vi "Coral Configuration.vi"() -> (2 "Algae Config":T2={"Setpoint Configs"=[{"Position Setpoint"=0.0, "Algae State"=enum."Idle", "Power Output"=0.0}, {"Position Setpoint"=5.0, "Algae State"=enum."Intake/Outtake", "Power Output"=-0.5}, {"Position Setpoint"=2.0, "Algae State"=enum."Intake/Outtake", "Power Output"=0.3}, {"Position Setpoint"=2.0, "Algae State"=enum."Stow", "Power Output"=-0.9}]}, 3 "Coral Config":T4={"Setpoint Configs"=[{"Scoring Setpoint"=enum."Trough", "Position Setpoint"=-9.0, "Trapezoid"=[-0.0, -40.0, -80.0, -120.0, -160.0, -200.0, -240.0, -280.0, -320.0, -360.0, -400.0, -440.0, -480.0, -520.0, -560.0, -600.0, -640.0, -680.0, -720.0, -760.0, -800.0, -840.0, -880.0, -920.0, -960.0, -1000.0, -960.0, -919.9999999999999, -879.9999999999999, -840.0000000000001, -800.0, -760.0, -720.0, -680.0, -639.9999999999999, -600.0000000000001, -560.0, -520.0, -480.0, -440.0, -399.9999999999999, -360.0000000000001, -320.0000000000001, -280.0, -240.0, -200.0, -159.9999999999999, -120.00000000000011, -80.00000000000011, -40.0, 0.0], "Score Power"=0.3}, {"Scoring Setpoint"=enum."L2", "Position Setpoint"=-9.7, "Trapezoid"=[], "Score Power"=0.5}, {"Scoring Setpoint"=enum."L3", "Position Setpoint"=-19.5, "Trapezoid"=[], "Score Power"=0.5}, {"Scoring Setpoint"=enum."L4", "Position Setpoint"=-34.9, "Trapezoid"=[], "Score Power"=0.9}, {"Scoring Setpoint"=enum."Default", "Position Setpoint"=0.0, "Trapezoid"=[], "Score Power"=0.0}]})   [LabVIEW 2023]
uses:
  Scoring Levels.ctl
  Algae Setpoint.ctl
panel:
  in  "Algae Intake Value":T2={"Setpoint Configs"=[{"Position Setpoint"=0.0, "Algae State"=enum."Idle", "Power Output"=0.0}, {"Position Setpoint"=5.0, "Algae State"=enum."Intake/Outtake", "Power Output"=-0.5}, {"Position Setpoint"=2.0, "Algae State"=enum."Intake/Outtake", "Power Output"=0.3}, {"Position Setpoint"=2.0, "Algae State"=enum."Stow", "Power Output"=-0.9}]}
  in  "Coral Config L3 Default":T4={"Setpoint Configs"=[{"Scoring Setpoint"=enum."Trough", "Position Setpoint"=-2.3, "Trapezoid"=[0.0, 80.0, 160.0, 240.0, 320.0, 400.0, 480.0, 560.0, 640.0, 720.0, 800.0, 880.0, 960.0, 960.0, 879.9999999999999, 800.0, 720.0, 639.9999999999999, 560.0, 480.0, 399.9999999999999, 320.0000000000001, 240.0, 159.9999999999999, 80.00000000000011, 0.0], "Score Power"=0.3}, {"Scoring Setpoint"=enum."L2", "Position Setpoint"=-3.5, "Trapezoid"=[0.0, 80.0, 160.0, 240.0, 320.0, 400.0, 480.0, 560.0, 640.0, 720.0, 800.0, 720.0000238418579, 640.0000238418579, 560.0000238418579, 480.0000238418578, 400.00002384185797, 320.0000238418579, 240.0000238418578, 160.0000238418579, 80.00002384185791, 0.0], "Score Power"=0.3}, {"Scoring Setpoint"=enum."L3", "Position Setpoint"=-7.0, "Trapezoid"=[], "Score Power"=0.2}, {"Scoring Setpoint"=enum."L4", "Position Setpoint"=-12.15, "Trapezoid"=[-0.0, -80.0, -160.0, -240.0, -320.0, -400.0, -480.0, -560.0, -640.0, -720.0, -800.0, -880.0, -960.0, -1040.0, -1120.0, -1200.0, -1280.0, -1247.6810359954834, -1167.6810359954834, -1087.6810359954834, -1007.6810359954833, -927.6810359954834, -847.6810359954834, -767.6810359954833, -687.6810359954835, -607.6810359954834, -527.6810359954833, -447.6810359954833, -367.68103599548317, -287.6810359954835, -207.6810359954834, -127.6810359954834, -47.6810359954834, 0.0], "Score Power"=0.9}]}
  in  "Ground Intake Coral":T2={"Setpoint Configs"=[{"Position Setpoint"=0.0, "Algae State"=enum."Idle", "Power Output"=0.0}, {"Position Setpoint"=8.5, "Algae State"=enum."Intake/Outtake", "Power Output"=-0.6}, {"Position Setpoint"=3.0, "Algae State"=enum."Intake/Outtake", "Power Output"=0.6}, {"Position Setpoint"=0.5, "Algae State"=enum."Stow", "Power Output"=-0.6}]}
  in  "Coral Config Trusted Values":T4={"Setpoint Configs"=[{"Scoring Setpoint"=enum."Trough", "Position Setpoint"=-9.0, "Trapezoid"=[-0.0, -40.0, -80.0, -120.0, -160.0, -200.0, -240.0, -280.0, -320.0, -360.0, -400.0, -440.0, -480.0, -520.0, -560.0, -600.0, -640.0, -680.0, -720.0, -760.0, -800.0, -840.0, -880.0, -920.0, -960.0, -1000.0, -960.0, -919.9999999999999, -879.9999999999999, -840.0000000000001, -800.0, -760.0, -720.0, -680.0, -639.9999999999999, -600.0000000000001, -560.0, -520.0, -480.0, -440.0, -399.9999999999999, -360.0000000000001, -320.0000000000001, -280.0, -240.0, -200.0, -159.9999999999999, -120.00000000000011, -80.00000000000011, -40.0, 0.0], "Score Power"=0.3}, {"Scoring Setpoint"=enum."L2", "Position Setpoint"=-9.7, "Trapezoid"=[], "Score Power"=0.5}, {"Scoring Setpoint"=enum."L3", "Position Setpoint"=-19.5, "Trapezoid"=[], "Score Power"=0.5}, {"Scoring Setpoint"=enum."L4", "Position Setpoint"=-34.9, "Trapezoid"=[], "Score Power"=0.9}, {"Scoring Setpoint"=enum."Default", "Position Setpoint"=0.0, "Trapezoid"=[], "Score Power"=0.0}]}
  # "L2:  -250 or -100 test\nL3: -450\nL4:-755"
  # "old values"
  # "-2.6"
  # "sp: 0.5"
  # "-4"
  # "sp: 0.5"
  # "-7.7"
  # "-600?"
  # "sp: 0.9"
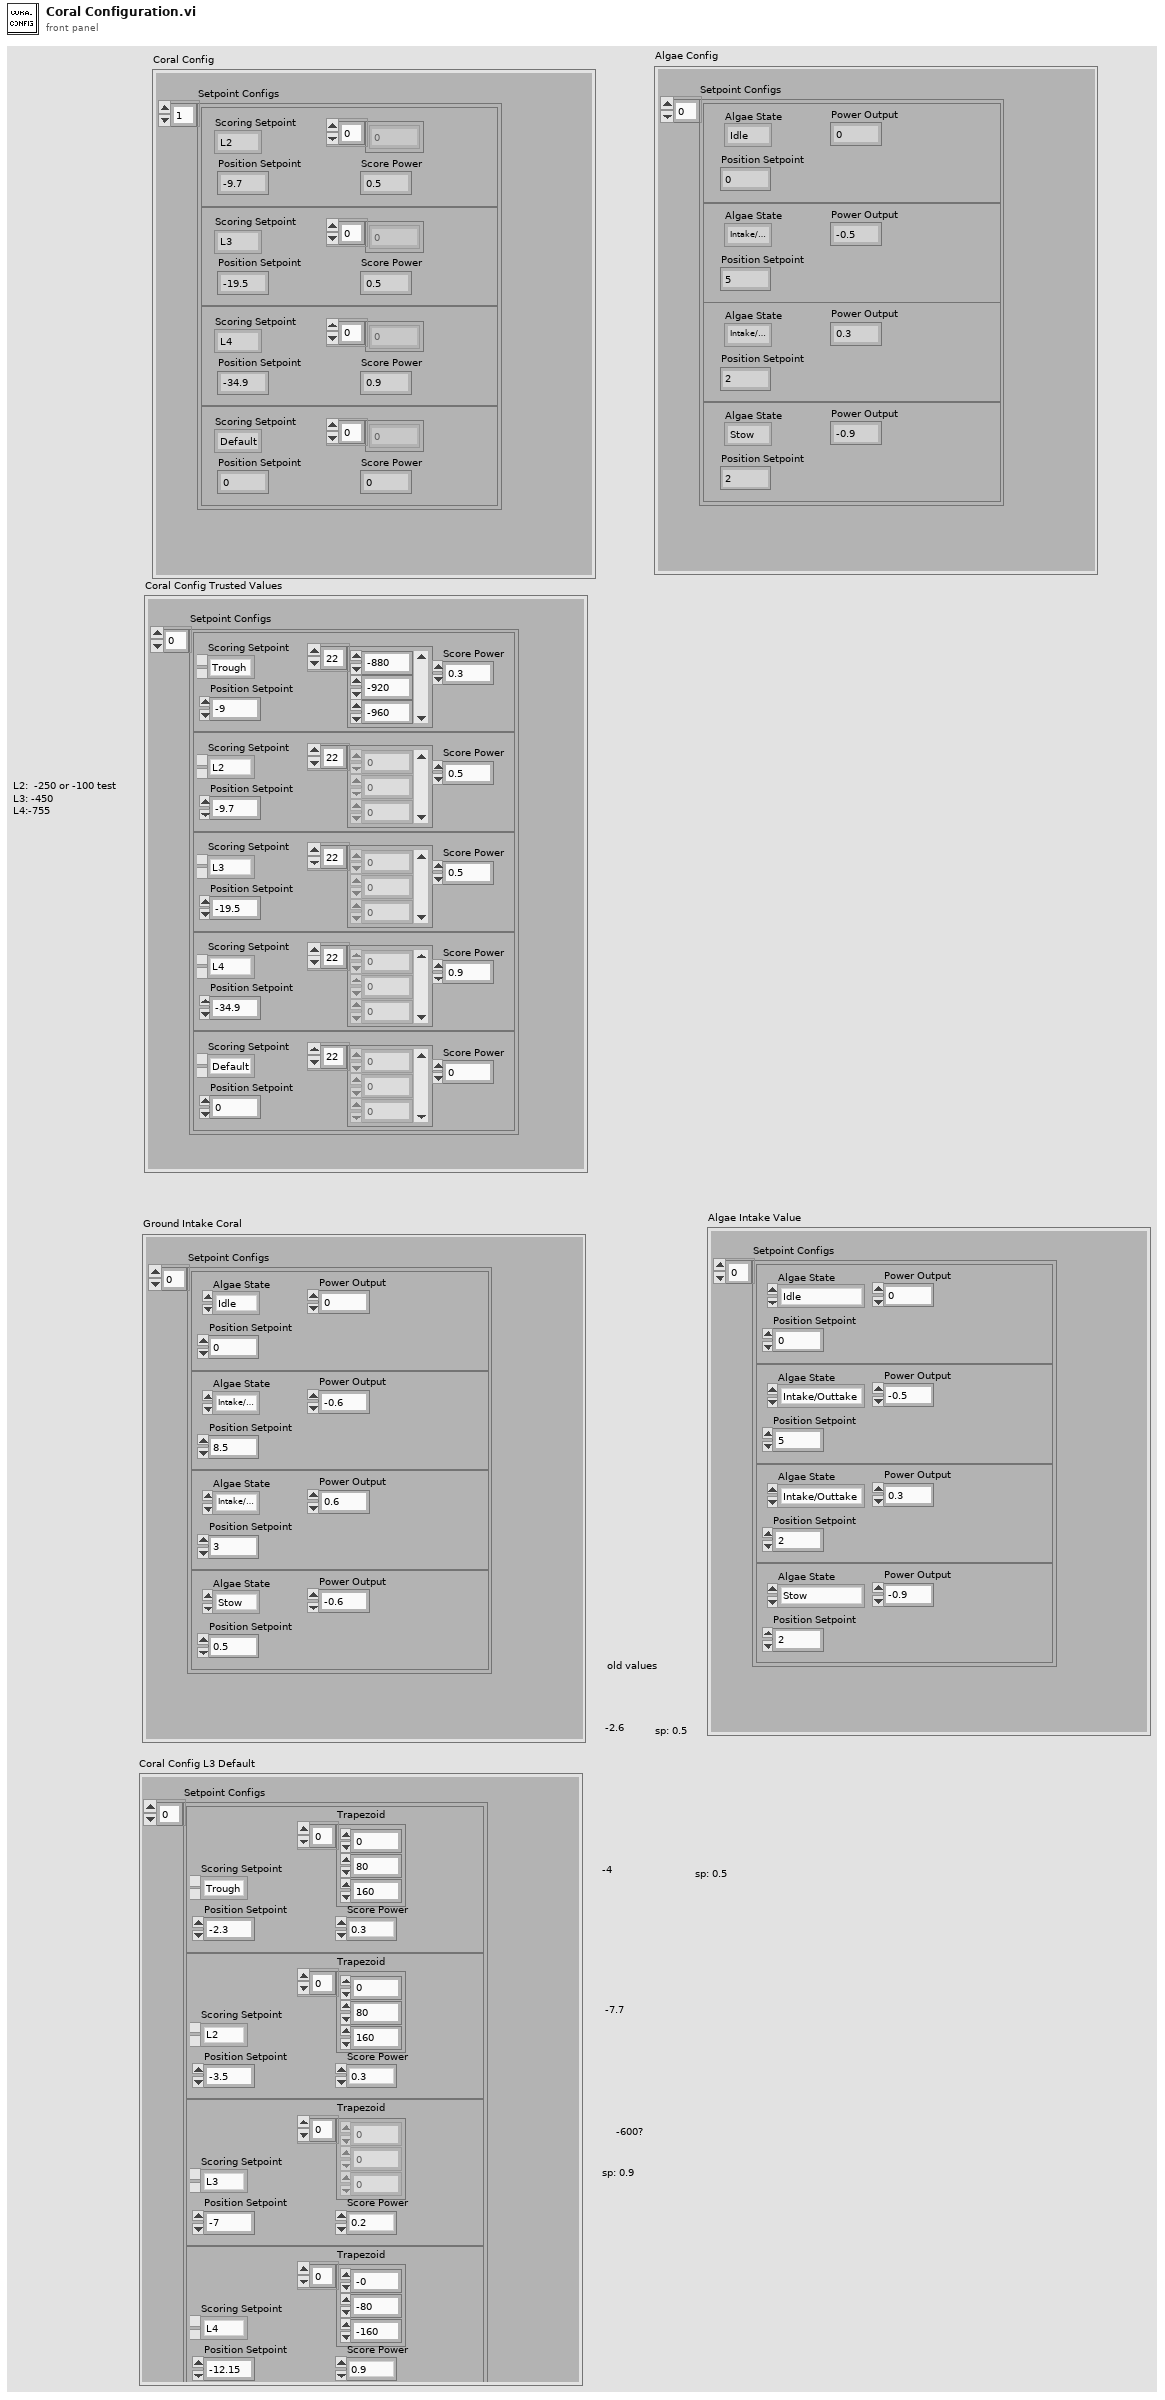
[diagram p1: front panel]
types:
  T1 = typedef "Algae Setpoint.ctl" = enum16{"Idle", "Stow", "Intake/Outtake"}
  T2 = cluster{"Setpoint Configs":cluster{"Position Setpoint":dbl, "Algae State":T1, "Power Output":dbl}[]}
  T3 = typedef "Scoring Levels.ctl" = enum16{"Trough", "L2", "L3", "L4", "Default"}
  T4 = cluster{"Setpoint Configs":cluster{"Scoring Setpoint":T3, "Position Setpoint":dbl, "Trapezoid":dbl[], "Score Power":dbl}[]}
  T5 = cluster{"Setpoint Configs":cluster{"Scoring Setpoint":T3, "Position Setpoint":dbl, "Trapezoid":dbl[]}[]}
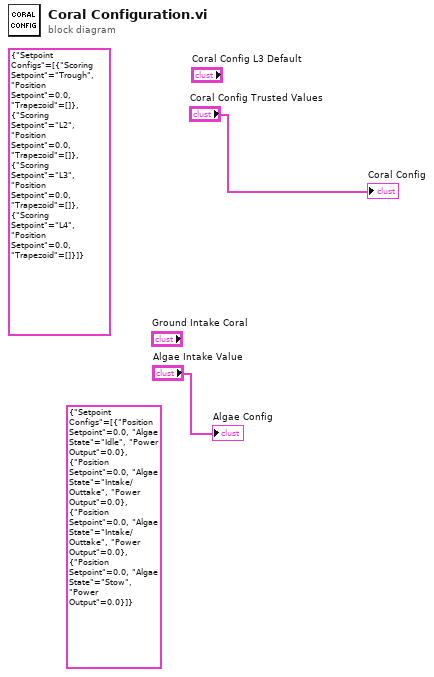
[diagram p0: block diagram]
diagram:
  (unwired) T2 {"Setpoint Configs"=[{"Position Setpoint"=0.0, "Algae State"=enum."Idle", "Power Output"=0.0}, {"Position Setpoint"=0.0, "Algae State"=enum."Intake/Outtake", "Power Output"=0.0}, {"Position Setpoint"=0.0, "Algae State"=enum."Intake/Outtake", "Power Output"=0.0}, {"Position Setpoint"=0.0, "Algae State"=enum."Stow", "Power Output"=0.0}]} ("Algae Config")
  (unwired) T5 {"Setpoint Configs"=[{"Scoring Setpoint"=enum."Trough", "Position Setpoint"=0.0, "Trapezoid"=[]}, {"Scoring Setpoint"=enum."L2", "Position Setpoint"=0.0, "Trapezoid"=[]}, {"Scoring Setpoint"=enum."L3", "Position Setpoint"=0.0, "Trapezoid"=[]}, {"Scoring Setpoint"=enum."L4", "Position Setpoint"=0.0, "Trapezoid"=[]}]} ("Coral Config")
  "Coral Config" <- "Coral Config Trusted Values"
  "Algae Config" <- "Algae Intake Value"
